vi "o3 Serial Packet Read.vi"(0 "VISA resource In":refnum<visa-resource-name>, 11 "error in":errorcluster) -> (4 "VISA resource Out":refnum<visa-resource-name>, 8 "Data Out":string, 15 "error out":errorcluster)   [LabVIEW 2014]
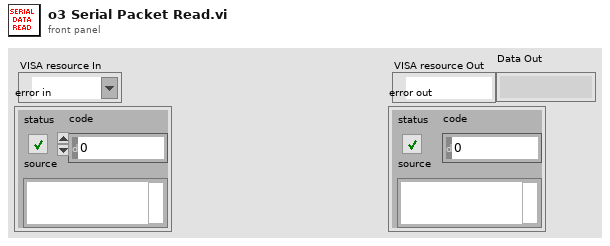
[diagram p1: front panel]
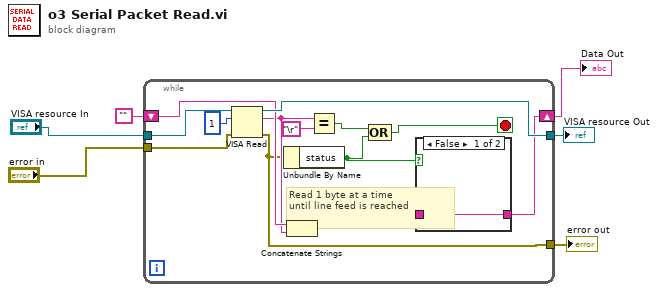
[diagram p0: block diagram]
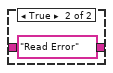
[diagram p2: hidden frame]
diagram:
  n1 = while {
    tunnel: [w19] -> w2
    tunnel: [w12] -> w1
    tunnel: "VISA resource In" -> [w18]
    tunnel: "error in" -> [w17]
    shift-right: [w10] -> w5
    shift-left: "" -> [w16]
    stop <- w7 stop-if-true
    # "Read 1 byte at a time \nuntil line feed is reached"
    n2 = VISA Read(VISA resource name=w18, byte count=u32 1, error in (no error)=w17) -> (VISA resource name out=w19:refnum<visa-resource-name>, read buffer=w15:string, error out=w12:errorcluster)  [unwired: 1 out]
    n3 = Unbundle By Name(w12) -> ("status"=w9:bool)
    n4 = Concatenate Strings(w16, w15) -> (w11:string)
    n5 = Equal?(x=w15, y="\r") -> (x = y?=w8:bool)
    n6 = Compound Arithmetic op=OR(w8, w9) -> (w7:bool)
    n7 = case shown="False" w9 {
      tunnel: w11 -> [w20 _]
      tunnel: [w20 "Read Error"] -> w10
      frame False {
      }
      frame True {
      }
    }
  }
  "VISA resource Out" <- w2
  "error out" <- w1
  "Data Out" <- w5
